vi "IFD SGL Image out.vi"(8 "error in (no error)":errorcluster, 10 "refnum in":refnum<file>, 11 "IFD in":refnum<class "IFD.lvclass">) -> (0 "error out":errorcluster, 2 "refnum out":refnum<file>)   [LabVIEW 2016, in "IFD.lvclass"]
uses:
  IFD.lvclass
  IFD.lvclass/IFD.ctl
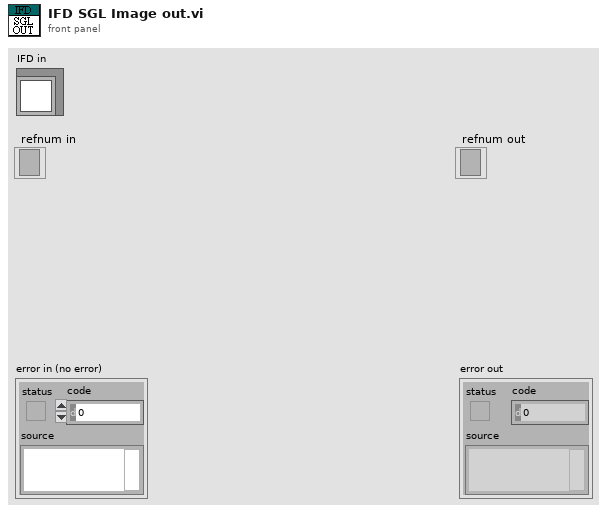
[diagram p1: front panel]
types:
  T1 = enum16{"big-endian, network order", "native, host order", "little-endian"}
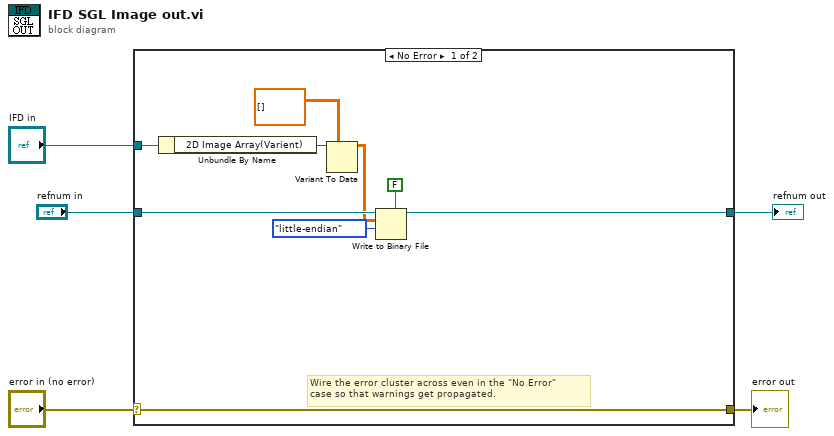
[diagram p0: block diagram]
diagram:
  n1 = case shown="No Error" "error in (no error)" {
    selector: "error in (no error)" -> [w14 w16]
    tunnel: [w14 w16] -> w4
    tunnel: "IFD in" -> [w13 _]
    tunnel: [w10 w15] -> w2
    tunnel: "refnum in" -> [w9 w15]
    frame No Error {
      # "Wire the error cluster across even in the \"No Error\"\ncase so that warnings get propagated."
      n2 = Unbundle By Name(w13) -> ("2D Image Array(Varient)"=w12:variant)
      n3 = Variant To Data(type=sgl[][] [], Variant=w12) -> (data=w7:sgl[][])  [unwired: 1 in, 1 out]
      n4 = Write to Binary File(file (use dialog)=w9, data=w7, 5:FALSE ("prepend array or string size? (T)"), 9:T1."little-endian" ("byte order (0:big-endian, network order)")) -> (refnum out=w10:refnum<file>)  [unwired: 2 in, 2 out]
    }
    frame Error {
    }
  }
  "error out" <- w4
  "refnum out" <- w2
